vi "Define 2D Heat PDE BC (Numeric).vi"(0 "PDE in":refnum<class "NI_PDE.lvclass">, 5 "Boundary Condition":dbl[][](array[numeric]), 7 "type":T2 items=["Dirichlet", "Neumann"], 9 "position":T1 items=["Start X", "End X", "Start Y", "End Y"], 11 "error in (no error)":errorcluster) -> (4 "PDE out":refnum<class "NI_PDE.lvclass">, 15 "error out":errorcluster)   [LabVIEW 2020, in "NI_PDE.lvlib"]
doc: "Defines the boundary condition of partial differential equations. You must manually select the polymorphic instance to use."
uses:
  <vilib>/gmath/NI_PDE.lvlib
  <vilib>/gmath/pde.llb/Common/PDE_BC Type.ctl
  <vilib>/gmath/pde.llb/PDEClass/NI_PDE.lvclass
  <vilib>/gmath/pde.llb/Common/PDE_BC Position 2D.ctl
  <vilib>/gmath/pde.llb/BCClass/BC_Evolut_2D_Numeric/NI_BC_Evolut_2D_Numeric.lvclass
  e:/builds/penguin/labview/branches/2020/dev/dist/vi.lib/gmath/pde.llb/BCClass/NI_BC.lvclass
  <vilib>/gmath/pde.llb/PDEClass/PDE_Heat_2D/NI_PDE_Heat_2D.lvclass
  e:/builds/penguin/labview/branches/2020/dev/dist/vi.lib/gmath/pde.llb/PDEClass/NI_PDE.lvclass
  <vilib>/gmath/pde.llb/BCClass/BC_Evolut_2D_Numeric/BC Data.ctl
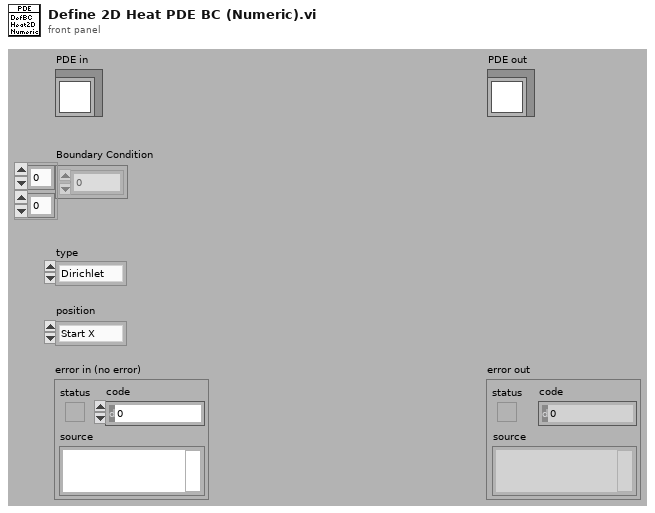
[diagram p1: front panel]
types:
  T1 = typedef "NI_PDE.lvlib/PDE_BC Position 2D.ctl" = i32
  T2 = typedef "NI_PDE.lvlib/PDE_BC Type.ctl" = i32
  T3 = typedef "NI_PDE.lvlib/NI_BC_Evolut_2D_Numeric.lvclass/BC Data.ctl" = cluster{"type":T2, "position":T1, "G":dbl[][]}
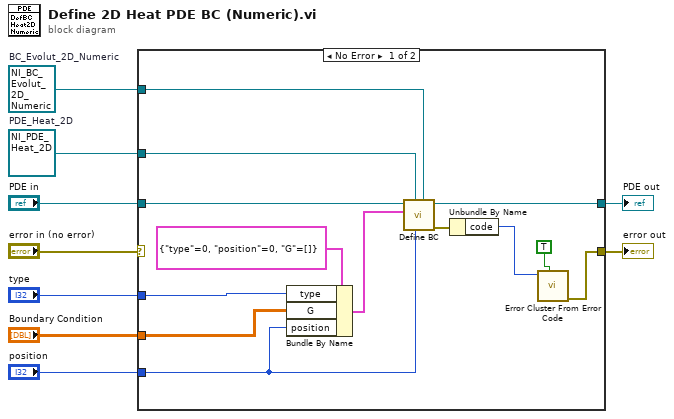
[diagram p0: block diagram]
diagram:
  w2 = refnum<class "NI_PDE_Heat_2D.lvclass"> refnum  # PDE_Heat_2D
  w1 = refnum<class "NI_BC_Evolut_2D_Numeric.lvclass"> refnum  # BC_Evolut_2D_Numeric
  n1 = case shown="No Error" "error in (no error)" {
    selector: "error in (no error)" -> [_ w24]
    tunnel: "PDE in" -> [w18 w23]
    tunnel: [w19 w23] -> w8
    tunnel: "position" -> [w12 _]
    tunnel: "Boundary Condition" -> [w14 _]
    tunnel: "type" -> [w15 _]
    tunnel: [w20 w24] -> w4
    tunnel: w2 -> [w11 _]
    tunnel: w1 -> [w10 _]
    frame No Error {
      n2 = Bundle By Name(cluster=T3 {"type"=0, "position"=0, "G"=[]} ("BC data"), "type"=w15, "G"=w14, "position"=w12) -> (w13:T3)
      n3 = call <vilib>:"Define BC.vi"("target BC"=w10, "index"=w12, "target PDE"=w11, "BC"=w13, "PDE in"=w18) -> ("error out"=w17:errorcluster, "PDE out"=w19:refnum<class "NI_PDE.lvclass">)  [unwired: 2 in, 3 out]
      n4 = Unbundle By Name(w17) -> ("code"=w22:i32)
      n5 = call <vilib>:"Error Cluster From Error Code.vi"("show call chain? (False)"=TRUE, "error code (0)"=w22) -> ("error out"=w20:errorcluster)  [unwired: 1 in, 6 out]
    }
    frame Error {
    }
  }
  "PDE out" <- w8
  "error out" <- w4
